vi "Fetch in 3Phase State.vi"(8 "error in":errorcluster, 9 "Fetch Type":u16(ring) items=["AC Voltage", "AC Current", "Real Power", "Apparent Power", "Pfactor Power", "Frequency", "Peak Current", "Peak Voltage", "Peak Plus Current", "Peak Minus Current", "THD", "Current THD", "Reactive Power"], 10 "Phase":enum16{"A", "B", "C", "ALL"}(ring), 11 "VISA resource name":refnum<visa-resource-name>) -> (0 "error out":errorcluster, 1 "Measurement":string, 3 "VISA resource name out":refnum<visa-resource-name>)   [LabVIEW 2015, in "IT-M7700.lvlib"]
doc: "Querys the actual value of the specified fetch for a desired channel.\n<b>Phase</b>\n0: A\n1: B\n2: C\n<b>Fetch Type</b>\n0:This command is used to read the Vrms voltage value.\n1:This command is used to read the Irms current value.\n2:This command is used to read the active power value.\n3:This command is used to read the apparent power value.\n4:This command is used to read the power factor value.\n5:This command is used to read the frequency value.\n6:This command is used to read the surge current value.\n7:This command is used to read the maximum voltage peak.\n8:This command is used to read the maximum positive peak current reading for A,B,C,ALL.\n9:This command is used to read the maximum negative peak current reading for A,B,C,ALL.\n10:This command is used to read the THD.\n11:This command is used to read the Current THD.\n12:This command is used to read the value of reactive power."
uses:
  <instrlib>/IT-M7700/IT-M7700.lvlib
panel:
  in  "Max Timeout":u32=10000
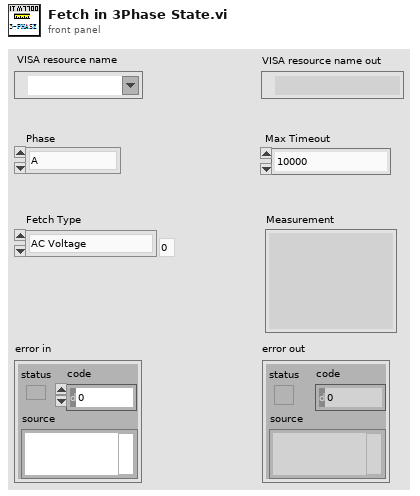
[diagram p1: front panel]
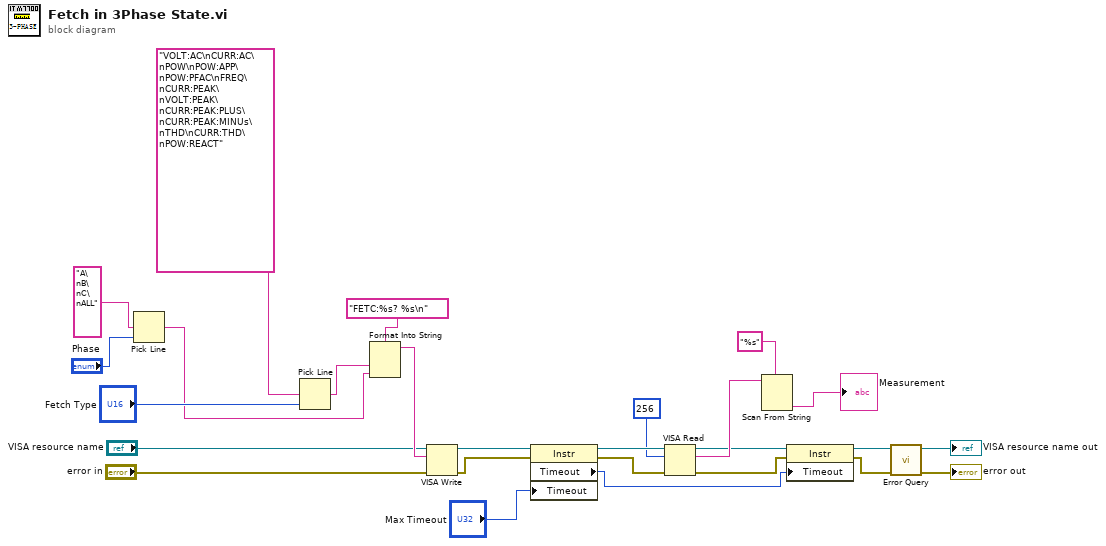
[diagram p0: block diagram]
diagram:
  n1 = Pick Line(multi-line string="A\nB\nC\nALL" ("多行字符串"), line index="Phase") -> (output string=w1:string)  [unwired: 1 in]
  n2 = Pick Line(multi-line string="VOLT:AC\nCURR:AC\nPOW\nPOW:APP\nPOW:PFAC\nFREQ\nCURR:PEAK\nVOLT:PEAK\nCURR:PEAK:PLUS\nCURR:PEAK:MINUs\nTHD\nCURR:THD\nPOW:REACT", line index="Fetch Type") -> (output string=w8:string)  [unwired: 1 in]
  n3 = Format Into String ("格式化写入字符串")(format string="FETC:%s? %s\n", w8, w1) -> (resulting string=w25:string)  [unwired: 2 in, 1 out]
  n4 = VISA Write(VISA resource name="VISA resource name", write buffer=w25, error in (no error)="error in") -> (VISA resource name out=w6:refnum<visa-resource-name>, error out=w5:errorcluster)  [unwired: 1 out]
  n5 = property class="Instr"(reference=w6, error in=w5, "Timeout"="Max Timeout") -> (reference out=w20:refnum<visa-resource-name>, error out=w19:errorcluster, "Timeout"=w4:u32)
  n6 = VISA Read(VISA resource name=w20, byte count=256, error in (no error)=w19) -> (VISA resource name out=w16:refnum<visa-resource-name>, read buffer=w24:string, error out=w7:errorcluster)  [unwired: 1 out]
  n7 = Scan From String(format string="%s", input string=w24) -> (output 1=→"Measurement":string)  [unwired: 3 in, 3 out]
  n8 = property class="Instr"(reference=w16, error in=w7, "Timeout"=w4) -> (reference out=w14:refnum<visa-resource-name>, error out=w13:errorcluster)
  n9 = call <instrlib>:"Error Query.vi"("error in"=w13, "VISA resource name"=w14) -> ("error out"=→"error out":errorcluster, "VISA resource name out"=→"VISA resource name out":refnum<visa-resource-name>)  [unwired: 6 in, 2 out]
